vi "Flock_LocalExceptionTemplate.vi"(8 "Error In":errorcluster, 11 "Process List":T1) -> (0 "Error Out":errorcluster)   [LabVIEW 2014]
uses:
  CentralProcessMessaging/Flock_Shared_CentralProcessMessaging.lvlib
  Flock_ErrorHandling.lvlib
  LocalProcessMessaging/Flock_Shared_LocalProcessMessaging.lvlib
  ProcessList.ctl
  Flock_Shared_Messaging.lvlib
panel:
  out "resulting string":string
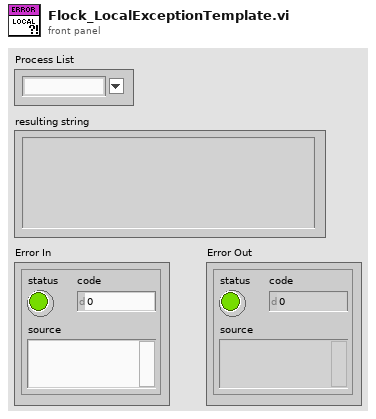
[diagram p1: front panel]
types:
  T1 = typedef "Flock_Shared_Messaging.lvlib/ProcessList.ctl" = string
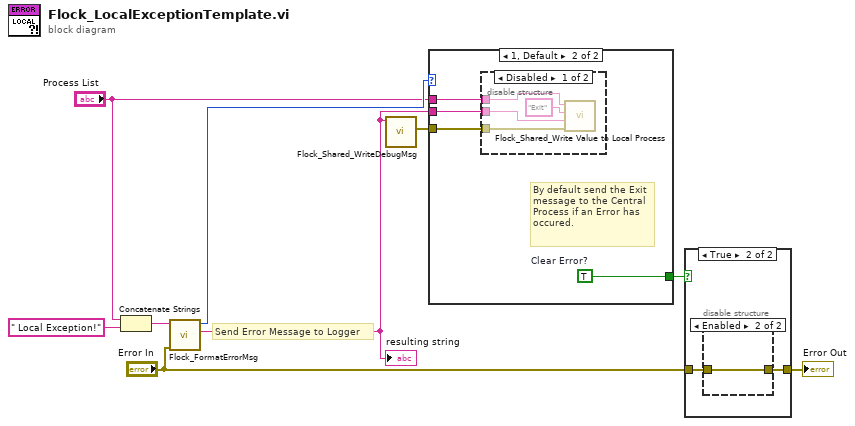
[diagram p0: block diagram]
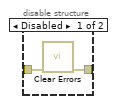
[diagram p3: hidden frame]
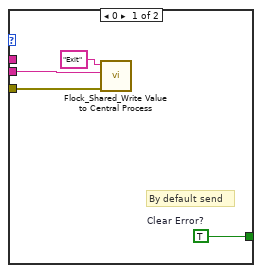
[diagram p4: hidden frame]
diagram:
  # "Send Error Message to Logger"
  n1 = Concatenate Strings("Process List", " Local Exception!" ("initial string")) -> (w1:string)
  n2 = call "Flock_FormatErrorMsg.vi"("error in (no error)"="Error In", "initial string"=w1) -> ("String"=w9:string, "code"=w8:i32)  [unwired: 8 in]
  "resulting string" <- w9
  n3 = call "Flock_Shared_WriteDebugMsg.vi"("Current Message Case"=w9) -> ("error out"=w4:errorcluster)  [unwired: 10 in]
  n4 = case shown="1, Default" w8 {
    tunnel: w9 -> [w12 w14]
    tunnel: [w11 w17] -> w7
    tunnel: w4 -> [w10 w16]
    tunnel: "Process List" -> [_ w15]
    frame 0 {
      w11 = TRUE  # Clear Error?
      # "By default send"
      n5 = call "Flock_Shared_Write Value to Central Process.vi"("error in (no error)"=w10, "Message Value"=w12, "Message Name"="Exit") -> ()  [unwired: 8 in, 1 out]
    }
    frame 1, Default {
      w17 = TRUE  # Clear Error?
      # "By default send the Exit message to the Central Process if an Error has occured."
      n6 = disable-structure shown="Disabled" {
        disable-tunnel: w16 -> [w21 _]
        disable-tunnel: w15 -> [w20 _]
        disable-tunnel: w14 -> [w18 _]
        frame Disabled {
          n7 = call "Flock_Shared_Write Value to Local Process.vi"("error in (no error)"=w21, "Message Value"=w18, "Message Name"="Exit", "Process List"=w20) -> ()  [unwired: 7 in, 1 out]
        }
        frame Enabled {
        }
      }
    }
  }
  n8 = case shown="True" w7 {
    tunnel: "Error In" -> [w22 w24]
    tunnel: [w22 w23] -> w5
    frame False {
    }
    frame True {
      n9 = disable-structure shown="Enabled" {
        disable-tunnel: w24 -> [w26 w27]
        disable-tunnel: [w25 w27] -> w23
        frame Disabled {
          n10 = call <vilib>:"Clear Errors.vi"("error in (no error)"=w26) -> ("error out"=w25:errorcluster)  [unwired: 5 in, 1 out]
        }
        frame Enabled {
        }
      }
    }
  }
  "Error Out" <- w5
